vi "test_Pointers.vi"() -> ()   [LabVIEW 2020]
uses:
  <vilib>/NI/Memory Manager/Classes/Pointer/Pointer.lvclass
  <vilib>/NI/Memory Manager/Classes/Pointer/Write Bool.vi
  <vilib>/NI/Memory Manager/Classes/Pointer/Read String.vi
  <vilib>/NI/Memory Manager/Classes/Pointer/Write 1D U64.vi
panel:
  out "dst 2":u8[](array[numeric])
  out "size":u64
  out "dst":T1
  out "error out":errorcluster
  out "return":i32
  in  "TY_FDX_UDP_BLOCK_WRITE_IN_MSG":T2(array[cluster])=[{"ul_UdpHandle"=1, "ul_ByteCount"=1, "pv_Data"=[3]}]
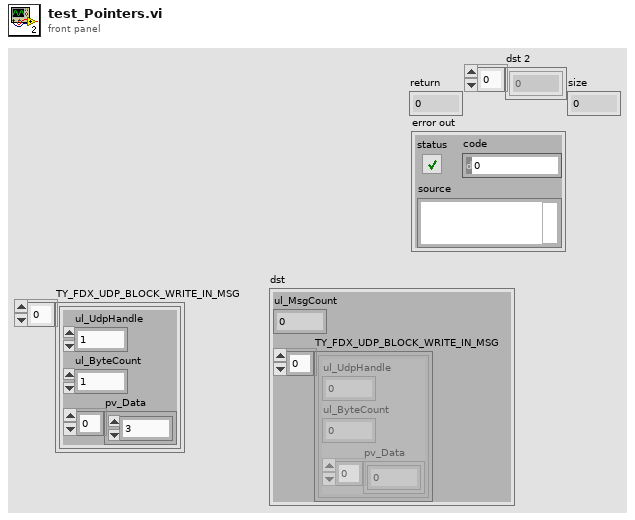
[diagram p1: front panel]
types:
  T1 = cluster{"ul_MsgCount":u32, "TY_FDX_UDP_BLOCK_WRITE_IN_MSG":cluster{"ul_UdpHandle":u32, "ul_ByteCount":u32, "pv_Data":u8[]}[]}
  T2 = cluster{"ul_UdpHandle":u32, "ul_ByteCount":u32, "pv_Data":u8[]}[]
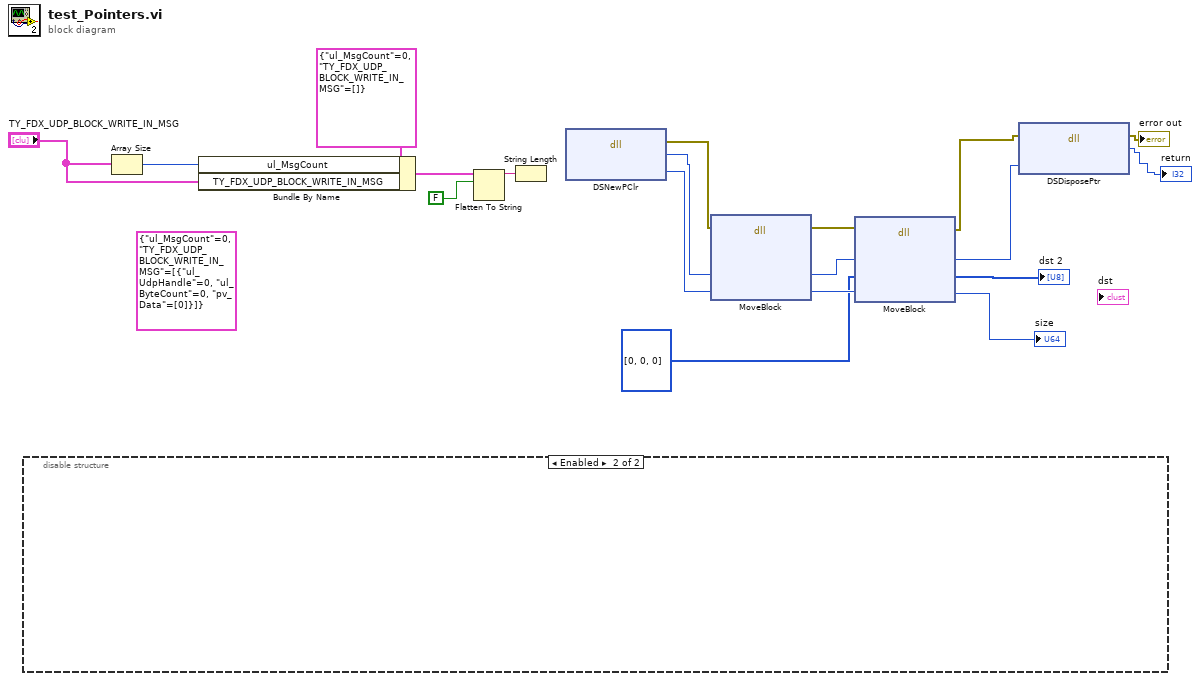
[diagram p0: block diagram]
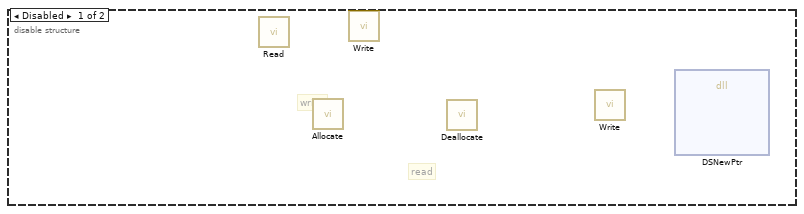
[diagram p2: hidden frame]
diagram:
  (unwired) T1 {"ul_MsgCount"=0, "TY_FDX_UDP_BLOCK_WRITE_IN_MSG"=[{"ul_UdpHandle"=0, "ul_ByteCount"=0, "pv_Data"=[0]}]} ("TY_FDX_UDP_BLOCK_WRITE_IN")
  n1 = disable-structure shown="Enabled" {
    frame Disabled {
      # "read"
      # "write"
      n2 = call-poly <vilib>:"Read.vi"() -> ()  [unwired: 8 in, 4 out]
      n3 = call <vilib>:"Allocate.vi"() -> ()  [unwired: 10 in, 2 out]
      n4 = call-poly <vilib>:"Write.vi"() -> ()  [unwired: 8 in, 4 out]
      n5 = call <vilib>:"Deallocate.vi"() -> ()  [unwired: 10 in, 2 out]
      n6 = call-poly <vilib>:"Write.vi"() -> ()  [unwired: 8 in, 4 out]
      n7 = dll-call lib="LabVIEW" fn="DSNewPtr"() -> ()  [unwired: 10 in, 2 out]
    }
    frame Enabled {
    }
  }
  n8 = Array Size(array="TY_FDX_UDP_BLOCK_WRITE_IN_MSG") -> (size(s)=w17:i32)
  n9 = Bundle By Name(cluster=T1 {"ul_MsgCount"=0, "TY_FDX_UDP_BLOCK_WRITE_IN_MSG"=[]} ("TY_FDX_UDP_BLOCK_WRITE_IN"), "ul_MsgCount"=w17, "TY_FDX_UDP_BLOCK_WRITE_IN_MSG"="TY_FDX_UDP_BLOCK_WRITE_IN_MSG") -> (w10:T1)
  n10 = Flatten To String(anything=w10, prepend array or string size? (T)=FALSE) -> (data string=w15:string)  [unwired: 2 in, 2 out]
  n11 = String Length(string=w15) -> ()  [unwired: 1 out]
  n12 = dll-call lib="LabVIEW" fn="DSNewPClr"() -> (error out=w9:errorcluster, "pointer"=w8:u64, "size"=w7:u64)  [unwired: 4 in, 1 out]
  n13 = dll-call lib="LabVIEW" fn="MoveBlock"(error in=w9, "dst"=w8, "size"=w7) -> (error out=w13:errorcluster, "dst"=w14:u64, "size"=w12:u64)  [unwired: 5 in, 1 out]
  n14 = dll-call lib="LabVIEW" fn="MoveBlock"(error in=w13, "src"=w14, "dst"=u8[] [0, 0, 0] ("pv_Data"), "size"=w12) -> (error out=w6:errorcluster, "src"=w5:u64, "dst"=→"dst 2":u8[], "size"=→"size":u64)  [unwired: 3 in, 1 out]
  n15 = dll-call lib="LabVIEW" fn="DSDisposePtr"(error in=w6, "pointer"=w5) -> (error out=→"error out":errorcluster, "return"=→"return":i32)  [unwired: 3 in, 1 out]
